vi "BASE.SaveConfig.vi"(8 "error in (no error)":errorcluster, 10 "config file path":path, 11 "BASE in":refnum<class "BASE.lvclass">) -> (0 "error out":errorcluster, 3 "BASE out":refnum<class "BASE.lvclass">)   [LabVIEW 2019, in "BASE.lvlib" / "BASE.lvclass"]
uses:
  BASE.lvclass
  BASE.lvclass/BASE.ctl
  <vilib>/Utility/config.llb/NI_LVConfig.lvlib
panel:
  out "class name":string
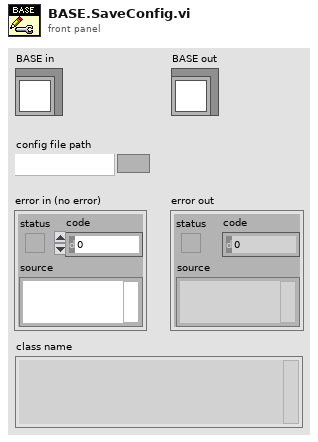
[diagram p1: front panel]
types:
  T1 = typedef "BASE.lvlib/BASE.lvclass/config--cluster.ctl" = cluster{"Config Path":path}
  T2 = typedef "NI_LVConfig.lvlib/Config Data RefNum.ctl" = refnum<k1>
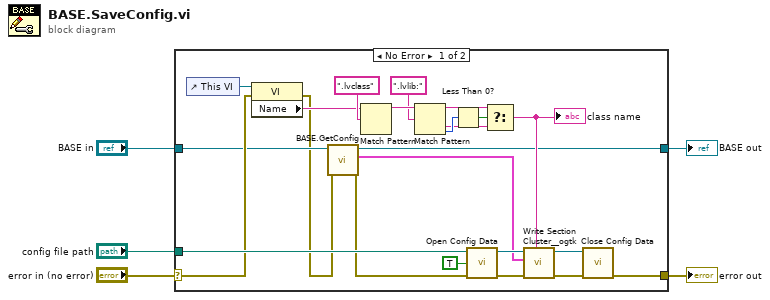
[diagram p0: block diagram]
diagram:
  n1 = case shown="No Error" "error in (no error)" {
    selector: "error in (no error)" -> [w22 w30]
    tunnel: [w25 w30] -> w4
    tunnel: [w9 w29] -> w2
    tunnel: "BASE in" -> [w10 w29]
    tunnel: "config file path" -> [w24 _]
    frame No Error {
      n2 = control-ref of="This VI"() -> (w23:refnum<vi>)
      n3 = property class="VI"(reference=w23, error in=w22) -> (error out=w7:errorcluster, "Name"=w13:string)  [unwired: 1 out]
      n4 = call "BASE.GetConfig.vi"("error in (no error)"=w7, "BASE in"=w10) -> ("error out"=w6:errorcluster, "Config"=w11:T1, "BASE out"=w9:refnum<class "BASE.lvclass">)  [unwired: 7 in]
      n5 = Match Pattern(string=w13, regular expression=".lvclass") -> (before substring=w19:string)  [unwired: 1 in, 3 out]
      n6 = Match Pattern(string=w19, regular expression=".lvlib:") -> (before substring=w17:string, after substring=w16:string, offset past match=w20:i32)  [unwired: 1 in, 1 out]
      n7 = Less Than 0?(x=w20) -> (x < 0?=w18:bool)
      n8 = call <vilib>:"Open Config Data.vi"("error in (no error)"=w6, "create file if necessary (T)"=TRUE, "configuration file path"=w24) -> ("error out"=w8:errorcluster, "refnum"=w28:T2)  [unwired: 6 in, 1 out]
      n9 = Select(t=w17, s=w18, f=w16) -> (s? t:f=w12:string)
      "class name" <- w12
      n10 = call <userlib>:"Write Section Cluster__ogtk.vi"("section (optional)"=w12, "error in (no error)"=w8, "Section Formatted Cluster"=w11, "refnum"=w28) -> ("error out"=w27:errorcluster, "dup refnum"=w26:T2)  [unwired: 6 in]
      n11 = call <vilib>:"Close Config Data.vi"("error in (no error)"=w27, "refnum"=w26) -> ("error out"=w25:errorcluster)  [unwired: 8 in, 1 out]
    }
    frame Error {
    }
  }
  "error out" <- w4
  "BASE out" <- w2
